vi "replaceDescriptionToken.vi"(8 "error in (no error)":errorcluster, 10 "Query In":string, 11 "Transaction in":refnum<class "Transaction.lvclass">) -> (0 "error out":errorcluster, 2 "Query Out":string, 3 "Transaction out":refnum<class "Transaction.lvclass">)   [LabVIEW 2018, in "Transaction.lvclass"]
uses:
  Transaction.lvclass
  Transaction.lvclass/Transaction.ctl
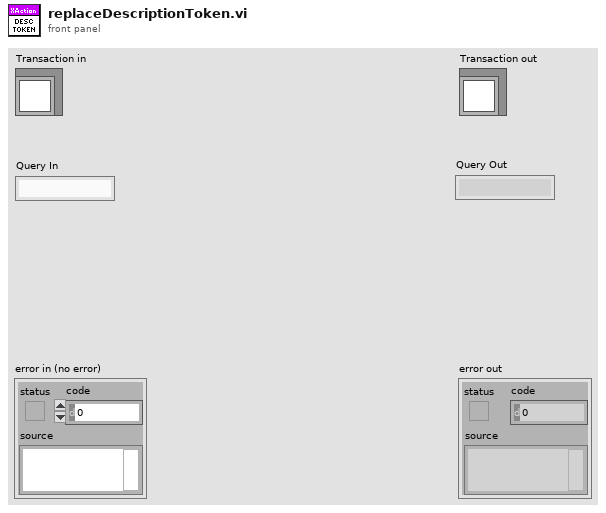
[diagram p1: front panel]
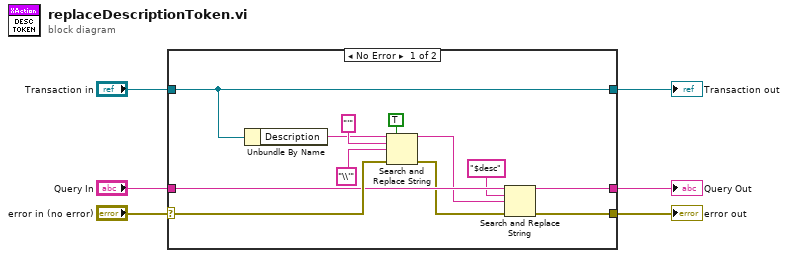
[diagram p0: block diagram]
diagram:
  n1 = case shown="No Error" "error in (no error)" {
    selector: "error in (no error)" -> [w13 w21]
    tunnel: [w10 w21] -> w5
    tunnel: [w18 w20] -> w3
    tunnel: "Transaction in" -> [w18 w20]
    tunnel: "Query In" -> [w12 w19]
    tunnel: [w11 w19] -> w1
    frame No Error {
      n2 = Unbundle By Name(w18) -> ("Description"=w14:string)
      n3 = Search and Replace String(replace all?=TRUE ("replace all? (F)"), input string=w14, search string="'", replace string="\\'", error in=w13) -> (result string=w8:string, error out=w9:errorcluster)  [unwired: 5 out]
      n4 = Search and Replace String(input string=w12, search string="$desc", replace string=w8, error in=w9) -> (result string=w11:string, error out=w10:errorcluster)  [unwired: 4 in, 2 out]
    }
    frame Error {
    }
  }
  "error out" <- w5
  "Transaction out" <- w3
  "Query Out" <- w1
